vi "Read Armed Response Synchronizer.vi"(8 "error in (no error)":errorcluster, 11 "Pulse Controller in":refnum<class "Pulse Controller.lvclass">) -> (0 "error out":errorcluster, 2 "Response Synchronizer.lvclass":refnum<class "Response Synchronizer.lvclass">, 3 "Pulse Controller out":refnum<class "Pulse Controller.lvclass">)   [LabVIEW 2021, in "Pulse Controller.lvclass"]
uses:
  Pulse Controller.lvclass
  Measurements/Response Synchronizer/Response Synchronizer.lvclass
  Pulse Controller.lvclass/Pulse Controller.ctl
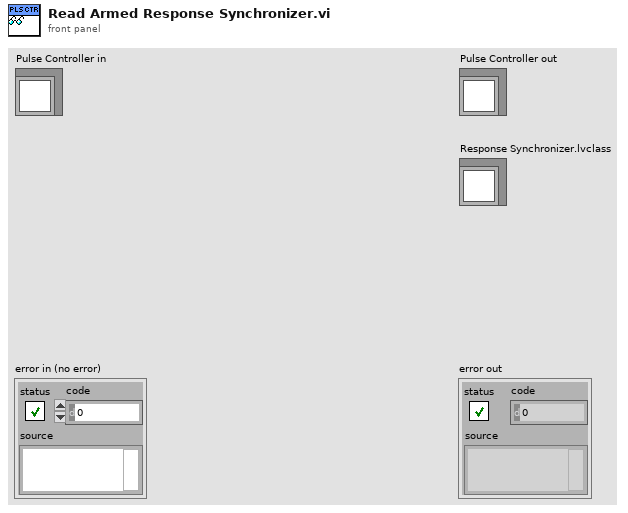
[diagram p1: front panel]
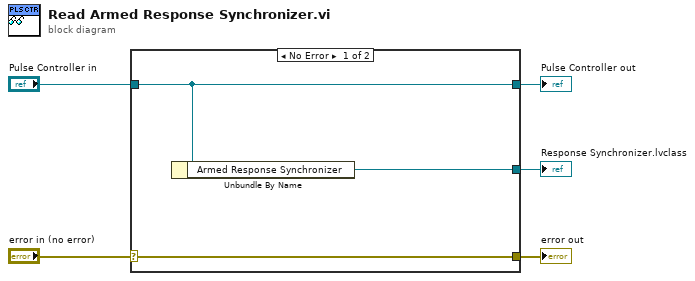
[diagram p0: block diagram]
diagram:
  n1 = case shown="No Error" "error in (no error)" {
    selector: "error in (no error)" -> [w8 w9]
    tunnel: [w8 w9] -> w4
    tunnel: [w7 w10] -> w2
    tunnel: "Pulse Controller in" -> [w7 w10]
    tunnel: [w6 _] -> w1
    frame No Error {
      n2 = Unbundle By Name(w7) -> ("Armed Response Synchronizer"=w6:refnum<class "Response Synchronizer.lvclass">)
    }
    frame Error {
    }
  }
  "error out" <- w4
  "Pulse Controller out" <- w2
  "Response Synchronizer.lvclass" <- w1
